vi "configurations to from repo cluster.vi"(8 "error in":errorcluster, 11 "configurations":refnum<class "CEF_serializable configuration.lvclass">[](array[class])) -> (0 "error out":errorcluster, 3 "from repo cluster":T1)   [LabVIEW 2023, in "CEF.lvlib" / "CEF_serializable node.lvclass"]
doc: "Copyright 2017 National Instruments Corporation\n\nLicensed under the Apache License, Version 2.0 (the \"License\"); you may not use this file except in compliance with the License. You may obtain a copy of the License at http://www.apache.org/licenses/LICENSE-2.0\nUnless required by applicable law or agreed to in writing, software distributed under the License is distributed on an \"AS IS\" BASIS, WITHOUT WARRANTIES OR CONDITIONS OF ANY KIND, either express or implied. See the License for the specific language governing permissions and limitations under the License."
uses:
  CEF_serializable node.lvclass
  Node/FromRepoCluster.ctl
  serializable configuration/CEF_serializable configuration.lvclass
  Node/CEF_Node.lvclass
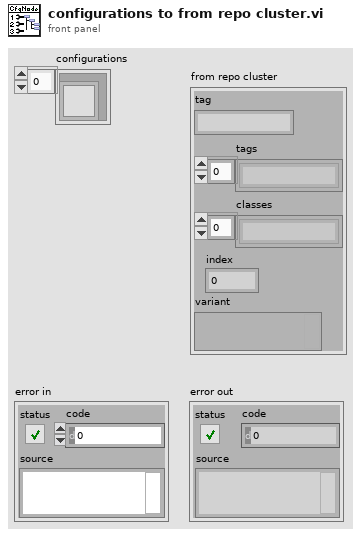
[diagram p1: front panel]
types:
  T1 = typedef "CEF.lvlib/CEF_Node.lvclass/FromRepoCluster.ctl" = cluster{"tag":string, "tags":string[], "classes":string[], "index":i32, "variant":variant}
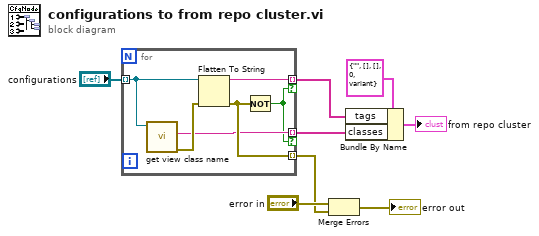
[diagram p0: block diagram]
diagram:
  n1 = for {
    tunnel: "configurations" -> [w14] mode=indexing
    tunnel: [w12] -> w6 mode=indexing
    tunnel: [w11] -> w1 mode=indexing if=w9
    tunnel: [w10] -> w2 mode=indexing if=w9
    n2 = call "get view class name.vi"("CEF_Configuration in"=w14) -> ("error out"=w13:errorcluster, "view class"=w11:string)  [unwired: 8 in, 1 out]
    n3 = Flatten To String(anything=w14, error in (no error)=w13) -> (data string=w10:string, error out=w12:errorcluster)  [unwired: 2 in, 1 out]
    n4 = Not(x=w12) -> (.not. x?=w9:bool)
  }
  n5 = Merge Errors("error in", w6) -> (→"error out":errorcluster)
  n6 = Bundle By Name(cluster=T1 {"tag"="", "tags"=[], "classes"=[], "index"=0, "variant"=variant} ("from repo cluster"), "tags"=w2, "classes"=w1) -> (→"from repo cluster":T1)
